vi "rs3 Advanced AE setpoint3.vi"(8 "error in (no error)":errorcluster, 10 "ST_AE_Control":cluster{"meanIntensitySetpoint":u32}, 11 "device in":u64) -> (0 "error out":errorcluster, 1 "error":u64, 3 "Dev out":u64)   [LabVIEW 2019, in "libRealSense3.lvlib"]
doc: "Sets the autoexposure setpoint."
uses:
  libRealSense3.lvlib
  realsense2.dll
panel:
  # "RS3 Adv. AE Setpoint"
  # "(C) 2017 Intel Corp.,  AGJ"
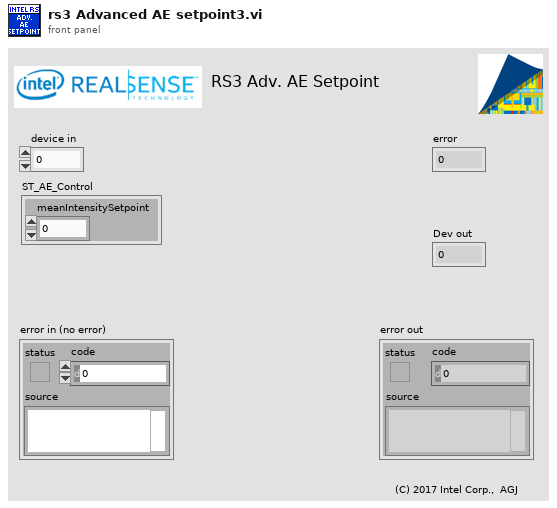
[diagram p1: front panel]
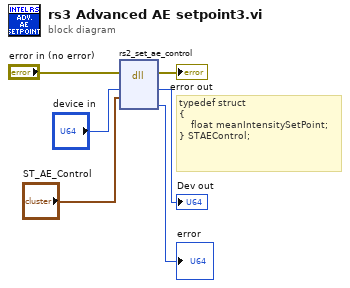
[diagram p0: block diagram]
diagram:
  # "typedef struct\n{\n    float meanIntensitySetPoint;\n} STAEControl;"
  n1 = dll-call lib="C:/SmartekVision/Projects/RS-D4-ETH/Software/RS-SDK/wrappers/labview/realsense2.dll" fn="rs2_set_ae_control"(error in="error in (no error)", "device"="device in", "AE control"="ST_AE_Control") -> (error out=→"error out":errorcluster, "device"=→"Dev out":u64, "error"=→"error":u64)  [unwired: 5 in, 1 out]
